vi "benchmarking_code.vi"() -> ()   [LabVIEW 2020]
panel:
  out "us/iteration":dbl
  in  "Iterations":i32
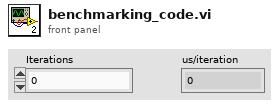
[diagram p1: front panel]
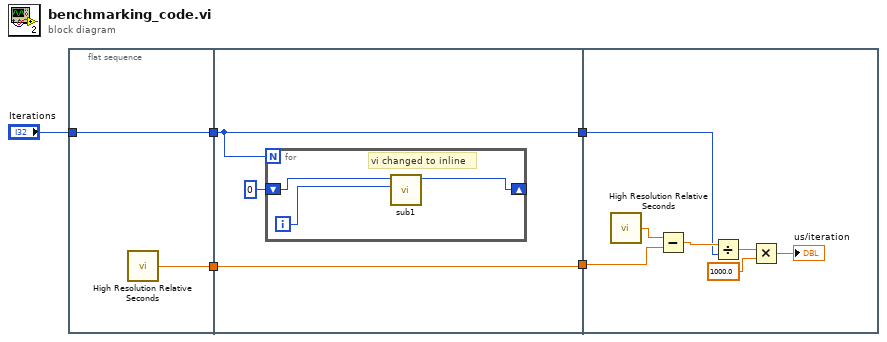
[diagram p0: block diagram]
diagram:
  n1 = flat-sequence {
    tunnel: [w7] -> w5
    tunnel: [w6] -> w4
    tunnel: "Iterations" -> [w6]
    tunnel: w5 -> [w10]
    tunnel: w4 -> [w8]
    tunnel: [w10] -> w2
    tunnel: [w8] -> w1
    tunnel: w2 -> [w20]
    tunnel: w1 -> [w17]
    frame #0 {
      n2 = call <vilib>:"High Resolution Relative Seconds.vi"() -> ("relative seconds"=w7:dbl)
    }
    frame #1 {
      n3 = for {
        N: w8 -> [_]
        shift-right: [w12] -> _
        shift-left: 0 -> [w11]
        i -> [w13]
        # "vi changed to inline"
        n4 = call "sub1.vi"("Numeric 3"=w13, "Numeric in"=w11) -> ("Numeric out"=w12:i32)  [unwired: 9 in]
      }
    }
    frame #2 {
      n5 = call <vilib>:"High Resolution Relative Seconds.vi"() -> ("relative seconds"=w19:dbl)
      n6 = Subtract(x=w19, y=w20) -> (x-y=w18:dbl)
      n7 = Divide(x=w18, y=w17) -> (x/y=w16:dbl)
      n8 = Multiply(x=w16, y=1000.0) -> (x*y=→"us/iteration":dbl)
    }
  }
